vi "PAM Job Setup TCP.vi"(7 "Error In":errorcluster {"code" format="%.0x"}, 9 "icListen #":i32, 10 "ID In":refnum<k5>) -> (0 "Error Out":errorcluster, 2 "Response":string, 3 "ID Out":refnum<k5>)   [LabVIEW 2020]
uses:
  PAM Sample Rate.vi
  PAM Library.lvlib
panel:
  out "Command 2":string
  out "Number":u32
  out "Command":string
  out "String":string
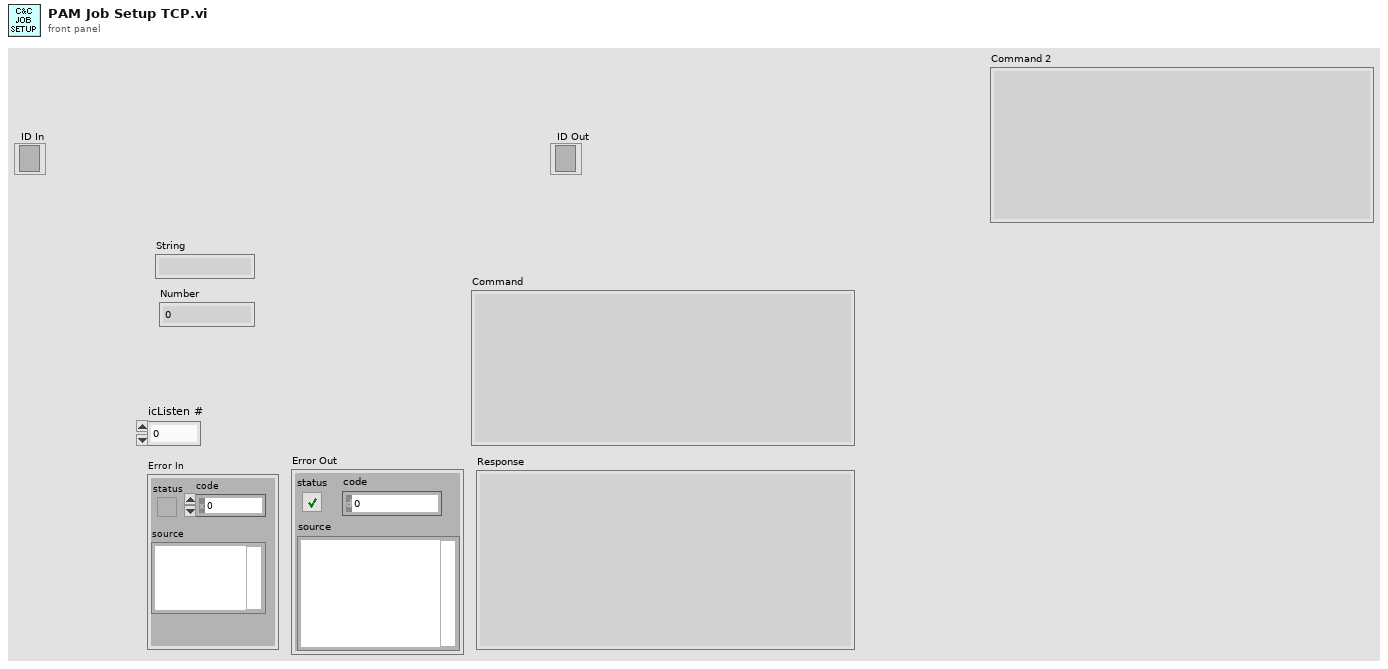
[diagram p1: front panel]
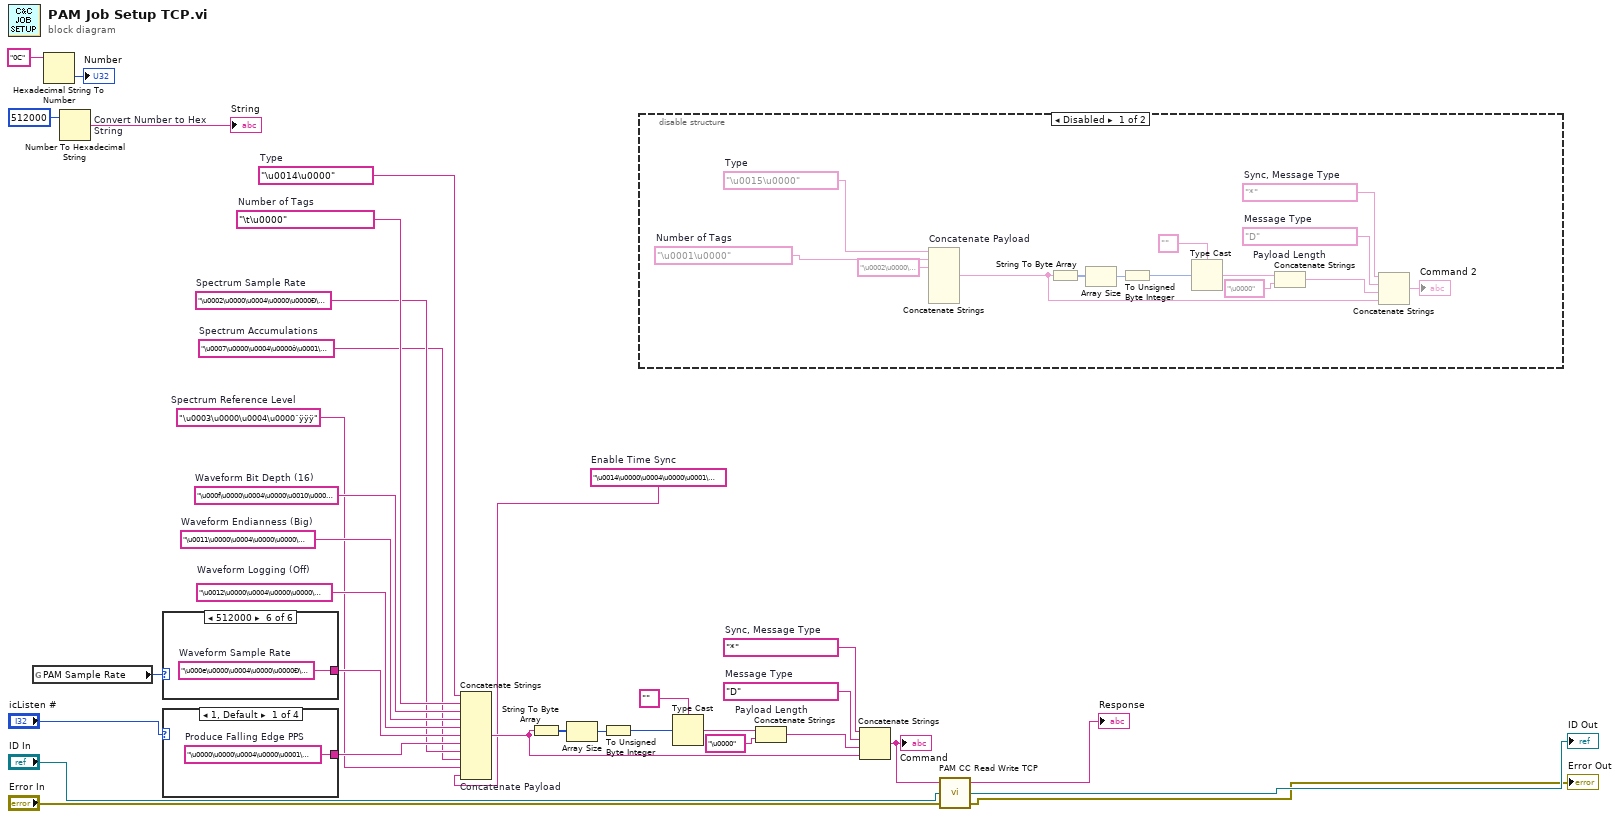
[diagram p0: block diagram]
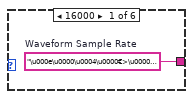
[diagram p3: hidden frame]
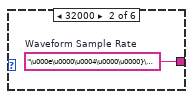
[diagram p4: hidden frame]
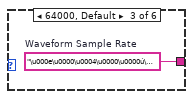
[diagram p5: hidden frame]
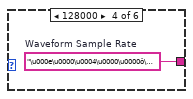
[diagram p6: hidden frame]
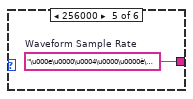
[diagram p7: hidden frame]
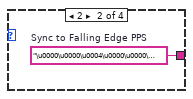
[diagram p8: hidden frame]
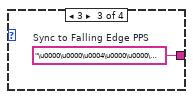
[diagram p9: hidden frame]
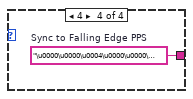
[diagram p10: hidden frame]
diagram:
  w1 = "\u0014\u0000\u0004\u0000\u0001\u0000\u0000\u0000"  # Enable Time Sync
  w3 = "\u0007\u0000\u0004\u0000ô\u0001\u0000\u0000"  # Spectrum Accumulations
  w4 = "\u0002\u0000\u0004\u0000\u0000Ð\u0007\u0000"  # Spectrum Sample Rate
  w2 = "\u0003\u0000\u0004\u0000ˆÿÿÿ"  # Spectrum Reference Level
  w18 = "\u0012\u0000\u0004\u0000\u0000\u0000\u0000\u0000"  # Waveform Logging (Off)
  w19 = "\u0011\u0000\u0004\u0000\u0000\u0000\u0000\u0000"  # Waveform Endianness (Big)
  w29 = "D"  # Message Type
  w6 = "\u0014\u0000"  # Type
  w5 = "\t\u0000"  # Number of Tags
  w28 = "\u000f\u0000\u0004\u0000\u0010\u0000\u0000\u0000"  # Waveform Bit Depth (16)
  w31 = "*"  # Sync, Message Type
  n1 = global read "PAM Sample Rate.vi" "PAM Sample Rate"() -> (w11:i32)
  n2 = Hexadecimal String To Number(string="0C") -> (number=→"Number":u32)  [unwired: 2 in, 1 out]
  n3 = Number To Hexadecimal String "Convert Number to Hex String"(2:512000) -> (0:→"String":string)  [unwired: 1 in]
  n4 = case shown="512000" w11 {
    tunnel: [w34 w35 w36 w37 w38 w39] -> w10
    frame 16000 {
      w34 = "\u000e\u0000\u0004\u0000€>\u0000\u0000"  # Waveform Sample Rate
    }
    frame 32000 {
      w35 = "\u000e\u0000\u0004\u0000\u0000}\u0000\u0000"  # Waveform Sample Rate
    }
    frame 64000, Default {
      w36 = "\u000e\u0000\u0004\u0000\u0000ú\u0000\u0000"  # Waveform Sample Rate
    }
    frame 128000 {
      w37 = "\u000e\u0000\u0004\u0000\u0000ô\u0001\u0000"  # Waveform Sample Rate
    }
    frame 256000 {
      w38 = "\u000e\u0000\u0004\u0000\u0000è\u0003\u0000"  # Waveform Sample Rate
    }
    frame 512000 {
      w39 = "\u000e\u0000\u0004\u0000\u0000Ð\u0007\u0000"  # Waveform Sample Rate
    }
  }
  n5 = case shown="1, Default" "icListen #" {
    tunnel: [w40 w41 w42 w43] -> w16
    frame 1, Default {
      w40 = "\u0000\u0000\u0004\u0000\u0001\u0000\u0000\u0000"  # Produce Falling Edge PPS
    }
    frame 2 {
      w41 = "\u0000\u0000\u0004\u0000\u0000\u0000\u0000\u0000"  # Sync to Falling Edge PPS
    }
    frame 3 {
      w42 = "\u0000\u0000\u0004\u0000\u0000\u0000\u0000\u0000"  # Sync to Falling Edge PPS
    }
    frame 4 {
      w43 = "\u0000\u0000\u0004\u0000\u0000\u0000\u0000\u0000"  # Sync to Falling Edge PPS
    }
  }
  n6 = Concatenate Strings "Concatenate Payload"(w6, w5, w28, w19, w18, w10, w16, w4, w3, w2, w1) -> (w27:string)
  n7 = String To Byte Array(string=w27) -> (unsigned byte array=w26:u8[])
  n8 = Array Size(array=w26) -> (size(s)=w21:i32)
  n9 = To Unsigned Byte Integer(number=w21) -> (unsigned 8bit integer=w20:u8)
  n10 = disable-structure shown="Disabled" {
    frame Disabled {
      w45 = "\u0001\u0000"  # Number of Tags
      w46 = "\u0015\u0000"  # Type
      w49 = "D"  # Message Type
      w48 = "*"  # Sync, Message Type
      n11 = Concatenate Strings "Concatenate Payload"(w46, w45, "\u0002\u0000\u0004\u0000" ("string")) -> (w50:string)  [unwired: 4 in]
      n12 = String To Byte Array(string=w50) -> (unsigned byte array=w51:u8[])
      n13 = Array Size(array=w51) -> (size(s)=w56:i32)
      n14 = To Unsigned Byte Integer(number=w56) -> (unsigned 8bit integer=w57:u8)
      n15 = Type Cast(type="", x=w57) -> (*(type *) &x=w55:string)
      n16 = Concatenate Strings "Payload Length"(w55, "\u0000") -> (w53:string)
      n17 = Concatenate Strings(w48, w49, w53, w50) -> (→"Command 2":string)
    }
    frame Enabled {
    }
  }
  n18 = Type Cast(type="", x=w20) -> (*(type *) &x=w22:string)
  n19 = Concatenate Strings "Payload Length"(w22, "\u0000") -> (w24:string)
  n20 = Concatenate Strings(w31, w29, w24, w27) -> (w30:string)
  "Command" <- w30
  n21 = call "PAM CC Read Write TCP.vi"("Error In"="Error In", "ID In"="ID In", "Command"=w30) -> ("Error Out"=→"Error Out":errorcluster, "ID Out"=→"ID Out":refnum<k5>, "Response"=→"Response":string)
